vi "Drive Controller.vi"(8 "error in":errorcluster) -> ()   [LabVIEW 2020]
doc: "This VI executes continuously carrying out the current operation and responding to updates or new operation requests. It will often contain the timing or control code that is difficult to place directly in TeleOp. This VI generally opens all sensors and motors and isolates the rest of the robot code from knowing implementation details of how the operations are carried out."
uses:
  <vilib>/Rock Robotics/WPI/Framework/Completion Status.ctl
  Drive Setpoints.ctl
  Drive Operations.ctl
  Support Code/submodules/bordeaux-pathinator/Bordeaux/Types/Single Cmd Info.ctl
  <vilib>/picture/picture.llb/imagedata.ctl
  <vilib>/Rock Robotics/WPI/ThirdParty/Phoenix-LabVIEW/Motor Controller/Controls/CTRE_Phoenix_MotorControl_ControlMode.ctl
  <vilib>/Platform/TimedLoop/XDataNode/timing_clust.ctl
  <vilib>/Platform/TimedLoop/XDataNode/nitl_modes.ctl
  <vilib>/Platform/TimedLoop/XDataNode/wakeup.ctl
  <vilib>/Rock Robotics/WPI/ThirdParty/Phoenix-LabVIEW/CANCoder/Get/CTRE_Phoenix_CANcoder_GetSensorData.vi
  <vilib>/Platform/TimedLoop/XDataNode/XDataNode.xnode
  <vilib>/Platform/TimedLoop/XDataNode/XDNodeRunTimeDep.lvlib
  7c524804-90ba-49ae-a8d8-e902cfb15891.vi
  Framework/Robot Global Data.vi
  03237a54-0aa6-442f-88f7-9e8753c34860.vi
  829c4970-17fc-441a-8aa9-59a5cf39e87e.vi
panel:
  out "size(s)":i32
  in  "IMU Correction  2":bool=TRUE
  out "Waveform Chart":dbl(graph)
  out "output cluster 2":T1
  out "output cluster":T2
  in  "teleop imu":bool
  in  "RESET CANCODERS -- TEST":bool
  in  "IMU Correction":bool=TRUE
  out "offsets":cluster{dbl, dbl, dbl, dbl}
  in  "pod radius":dbl=1.166667
  in  "Interactive Values":T3
  in  "Buttons":cluster{"Execute Cmd":bool, "Abort Cmd":bool}
  out "Command Timing":cluster{"Start Time (ms)":u32, "Iterations":i32}
  out "Status":T7
  out "Current\nCmd":string
  # "Tip: The graph shows the motor setpoints. It may also be helpful to observe inputs and sensor values.\nYou may also want to display tuning or debugging controls."
  # "Interactive Command: You may fill in the settings for a command\nand schedule it with the Execute button. You can observe and abort\nany command while fine tuning the code for the controller."
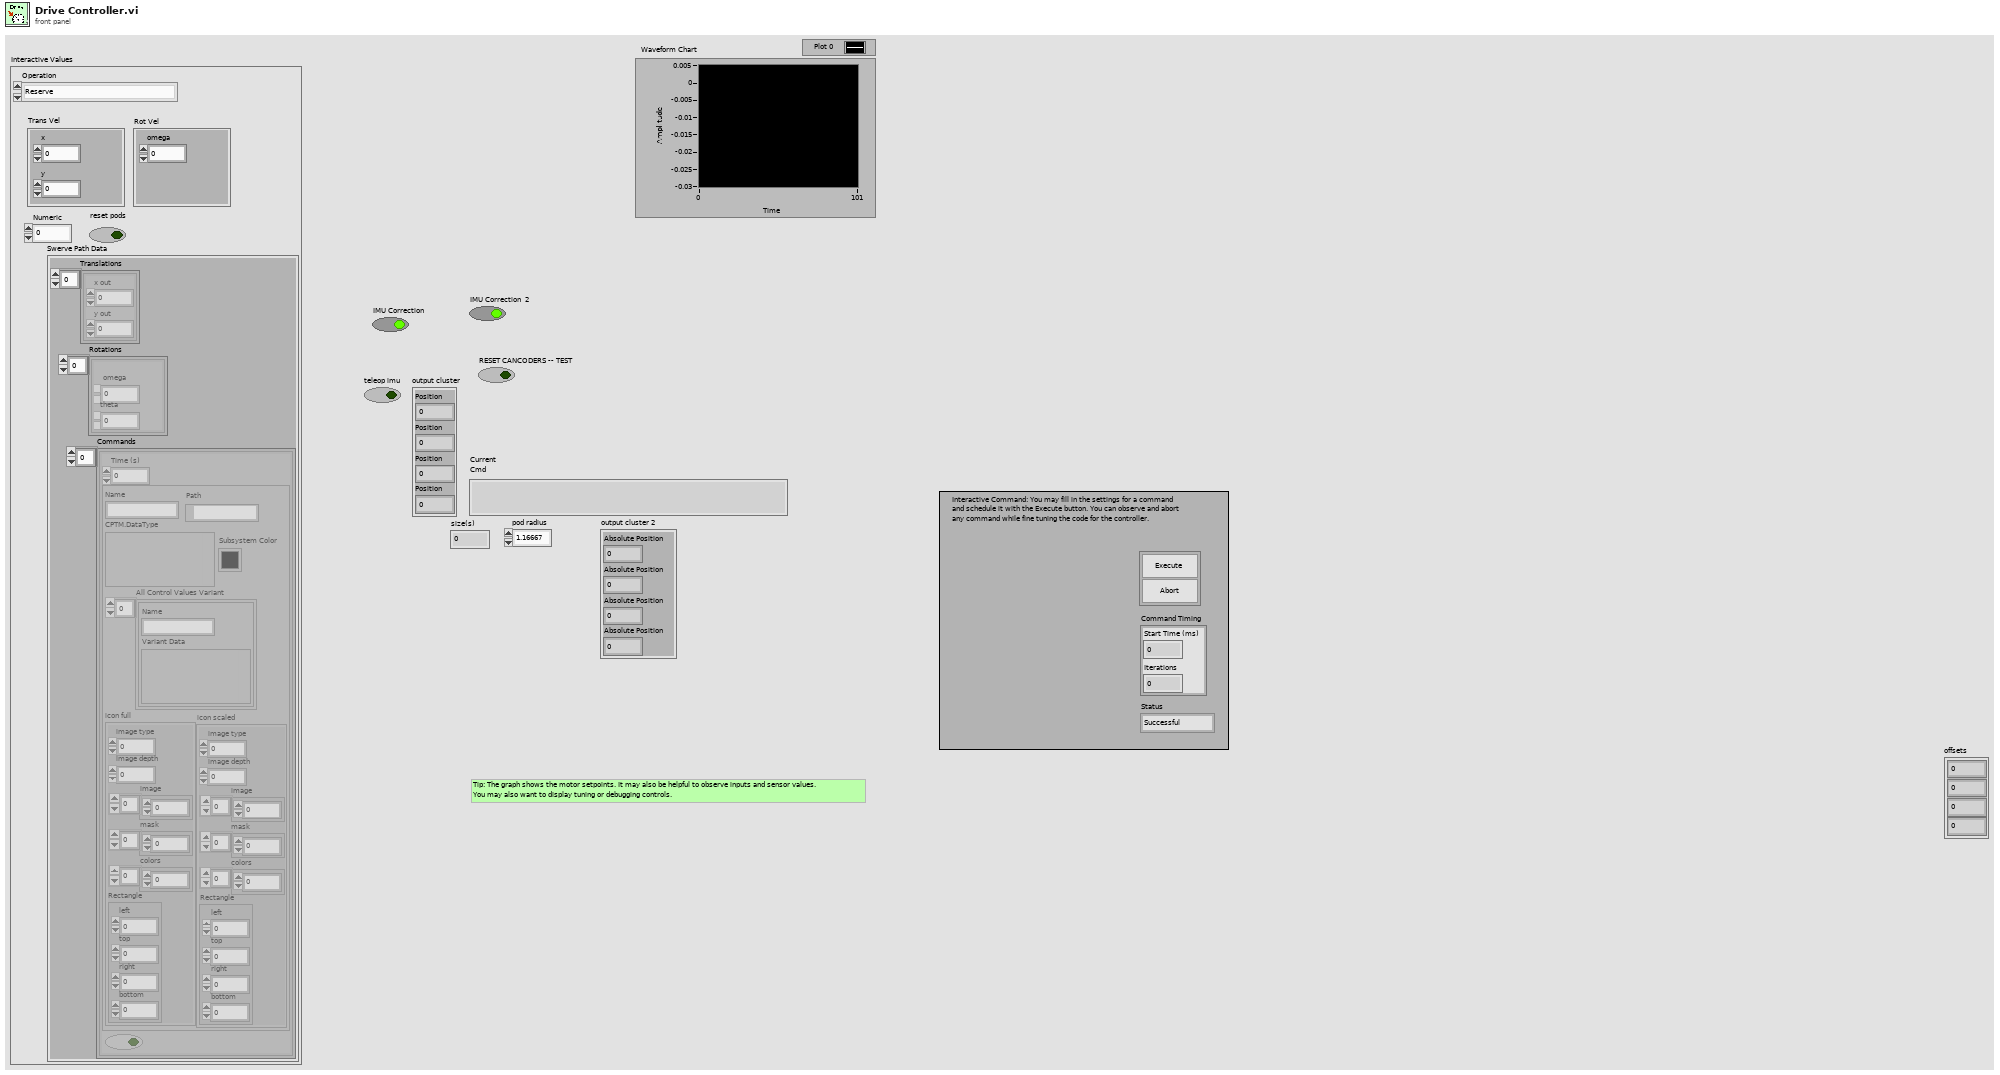
[diagram p1: front panel]
types:
  T1 = cluster{"Absolute Position":dbl, "Absolute Position":dbl, "Absolute Position":dbl, "Absolute Position":dbl}
  T2 = cluster{"Position":dbl, "Position":dbl, "Position":dbl, "Position":dbl}
  T3 = typedef "Drive Setpoints.ctl" = cluster{"Operation":T4, "Trans Vel":cluster{"x":dbl, "y":dbl}, "Rot Vel":cluster{"omega":dbl}, "Swerve Path Data":cluster{"Translations":cluster{"x out":dbl, "y out":dbl}[], "Rotations":cluster{"omega":dbl, "theta":dbl}[], "Commands":cluster{"Time (s)":dbl, T5, bool}[]}, "reset pods":bool, "Numeric":dbl}
  T4 = typedef "Drive Operations.ctl" = enum16{"Reserve", "Read Current", "Immediate", "Calibrate", "Play Path", "Immediate MM", "Set Schtuff"}
  T5 = typedef "Single Cmd Info.ctl" = cluster{"Name":string, "CPTM.DataType":variant, "All Control Values Variant":cluster{"Name":string, "Variant Data":variant}[], "icon full":T6, "icon scaled":T6, "Path":path, "Subsystem Color":u32}
  T6 = typedef "imagedata.ctl" = cluster{"image type":i32, "image depth":i32, "image":u8[], "mask":u8[], "colors":u32[], "Rectangle":cluster{"left":i16, "top":i16, "right":i16, "bottom":i16}}
  T7 = typedef "Completion Status.ctl" = enum16{"Successful", "Aborted", "Incomplete"}
  T8 = cluster{"LF ID":u8, "LB ID":u8, "RF ID":u8, "RB ID":u8}
  T9 = cluster{"LF radius":dbl[], "LB radius":dbl[], "RF radius":dbl[], "RB radius":dbl[]}
  T10 = typedef "Command Status Info.ctl" = cluster{"Name":string, "Status":T7, "notifier out":T11}
  T11 = typedef "Completion Notifier.ctl" = refnum<notifier>
  T12 = cluster{"SubSystem Data":T3, cluster{"Start Time (ms)":u32, "Iterations":i32}, cluster{"Command Info":T10, "Description":string, "Default Command":T3, "queue out":refnum<queue>, "Subsystem Name":string}}
  T13 = typedef "CTRE_Phoenix_MotorControl_BufferedTrajectoryPointStream_DeviceRef.ctl" = cluster{"Handle":u64, "Library Path":path}
  T14 = cluster{"BufferedTrajectoryPointStream_DevRef":T13, "BufferedTrajectoryPointStream_DevRef":T13, "BufferedTrajectoryPointStream_DevRef":T13, "BufferedTrajectoryPointStream_DevRef":T13}
  T15 = typedef "WPI_MotorControlDeviceRef.ctl" = cluster{"DeviceStatus":errorcluster, "Type":T16, "PWM":cluster{"PWM Channel":T17, "DeadBand":T18}, "CAN":cluster{"Device Number":u8, "SetOutput VI Ref":variant, "GetOutput VI Ref":variant, "Enable VI Ref":variant, "Disable VI Ref":variant, "Data":variant}, "Invert":bool, "DIO PWM":cluster{"PWM \"Enable\" Channel":T17, "DIOChannel":T19, "PWM Rate":dbl}}
  T16 = typedef "WPI_MotorControlType.ctl" = enum16{"PWM", "CAN", "DIO PWM"}
  T17 = typedef "FPGA_DIOPWMChannel.ctl" = enum8{"PWM 0", "PWM 1", "PWM 2", "PWM 3", "PWM 4", "PWM 5", "PWM 6", "PWM 7", "PWM 8", "PWM 9", "PWM MXP 0", "PWM MXP 1", "PWM MXP 2", "PWM MXP 3", "PWM MXP 4", "PWM MXP 5", "PWM MXP 6", "PWM MXP 7", "PWM MXP 8", "PWM MXP 9", "Invalid"}
  T18 = typedef "WPI_PWMDeadband.ctl" = cluster{"Name":string, "maxPositivePwm":i32, "minPositivePwm":i32, "centerPwm":i32, "maxNegativePwm":i32, "minNegativePwm":i32, "angularRange":u16}
  T19 = typedef "FPGA_DIOChannel.ctl" = enum8{"DIO 0", "DIO 1", "DIO 2", "DIO 3", "DIO 4", "DIO 5", "DIO 6", "DIO 7", "DIO 8", "DIO 9", "DIO MXP 0", "DIO MXP 1", "DIO MXP 2", "DIO MXP 3", "DIO MXP 4", "DIO MXP 5", "DIO MXP 6", "DIO MXP 7", "DIO MXP 8", "DIO MXP 9", "DIO MXP 10", "DIO MXP 11", "DIO MXP 12", "DIO MXP 13", "DIO MXP 14", "DIO MXP 15", "SPI Port CS1", "SPI Port CS2", "SPI Port CS3", "SPI Port MISO", "SPI Port MOSI", "Invalid"}
  T20 = cluster{"PhoenixMotorControlDevRef":T15, "PhoenixMotorControlDevRef":T15, "PhoenixMotorControlDevRef":T15, "PhoenixMotorControlDevRef":T15}
  T21 = typedef "ADIS16470 Device Reference.ctl" = cluster{"DevStatus":errorcluster, "Hardware Config":T22, "Calibration Complete":refnum<notifier>, "Status Reference":refnum<data-value>, "Position Reference":refnum<data-value>, "Velocity Reference":refnum<data-value>, "Sychronous Process VI":T25, "Cmd FIFO":refnum<k33>, "Source":T26, "Data FIFO":refnum<k33>, "Calibration Time (ms)":u32}
  T22 = typedef "ADIS16470 Hardware Configuration.ctl" = cluster{"SPI Clock Rate (Hz)":dbl, "IMU SPI Mode (3)":T23, "IMU Reset Pin":T19, "IMU SPI Bus":T24, "IMU Data Ready Pin":T19, "Stall Config":cluster{"Pow2BytesPerRead":u8, "StallTicks":u16, "CsToSclkTicks":u8}}
  T23 = typedef "WPI_SPIMode.ctl" = enum16{"Mode 0 (Clk Idle Low,Sample on Leading)", "Mode 1 (Clk Idle Low,Sample on Trailing)", "Mode 2 (Clk Idle High,Sample on Leading)", "Mode 3 (Clk Idle High,Sample on Trailing)"}
  T24 = typedef "spi_bus.ctl" = enum16{"SPI On-Board, CS0", "SPI On-Board, CS1", "SPI On-Board, CS2", "SPI On-Board, CS3", "SPI MXP", "Invalid"}
  T25 = typedef "ADIS16470 Process.ctl" = refnum<vi>
  T26 = typedef "FPGA_CounterEncoderSourceConvertionLVSourceType.ctl" = cluster{"DevStatus":errorcluster, "AnalogTriggerMode?":bool, "DigitalMode":cluster{"DIO Channel":T27}, "AnalogTriggerMode":cluster{"AnalogTriggerIndex":T28, "OutputType":T29}}
  T27 = typedef "FPGA_DIODigitalSourceChannel.ctl" = enum8{"DIO 0", "DIO 1", "DIO 2", "DIO 3", "DIO 4", "DIO 5", "DIO 6", "DIO 7", "DIO 8", "DIO 9", "DIO MXP 0", "DIO MXP 1", "DIO MXP 2", "DIO MXP 3", "DIO MXP 4", "DIO MXP 5", "DIO MXP 6", "DIO MXP 7", "DIO MXP 8", "DIO MXP 9", "DIO MXP 10", "DIO MXP 11", "DIO MXP 12", "DIO MXP 13", "DIO MXP 14", "DIO MXP 15", "SPI Port CS1", "SPI Port CS2", "SPI Port CS3", "SPI Port MISO", "SPI Port MOSI", "Disabled"}
  T28 = typedef "FPGA_AnalogTriggerIndex.ctl" = enum8{"Trig 0", "Trig 1", "Trig 2", "Trig 3", "Trig 4", "Trig 5", "Trig 6", "Trig 7", "Invalid"}
  T29 = typedef "FPGA_AnalogTriggerOutType.ctl" = enum16{"InWindow", "TriggerState", "Rising", "Falling"}
  T30 = typedef "CTRE_Phoenix_CANcoder_DeviceRef.ctl" = cluster{"DeviceStatus":errorcluster, "Device Number":u8, "Handle":u64, "UsageFrame":u32, "Library Path":path}
  T31 = cluster{"CTRE_CANcoder_DeviceRef":T30, "CTRE_CANcoder_DeviceRef":T30, "CTRE_CANcoder_DeviceRef":T30, "CTRE_CANcoder_DeviceRef":T30}
  T32 = typedef "XDNodeRunTimeDep.lvlib/timing_clust.ctl" = cluster{"Expected End [f-1]":u64, "Actual End [f-1]":u64, "Finished Late? [f-1]":bool, "Expected End [i-1]":u64, "Actual End [i-1]":u64, "Finished Late? [i-1]":bool, "Expected Start [i]":u64, "Actual Start [i]":u64, "Expected Start [f]":u64, "Actual Start [f]":u64, "Source Name":string, "Structure Name":string, "Period":i64, "Deadline":i64, "Offset":i64, "Start":i64, "Priority":i32, "Timeout":i32, "Mode":T33, "Wakeup Reason":T34, "Error":errorcluster, "Source Type":string, "Secondary Source Type":string, "Global End Time":u64, "Global Start Time":u64, "Frame Duration":u64, "Iteration Duration":u64, "Assigned CPU":i32, "I/O Scan Engine Mode":u32}
  T33 = typedef "XDNodeRunTimeDep.lvlib/nitl_modes.ctl" = enum32{"No Change", "Process missed periods, maintain original phase", "Discard missed periods, maintain original phase", "Process missed periods, ignore original phase", "Discard missed periods, ignore original phase"}
  T34 = typedef "XDNodeRunTimeDep.lvlib/wakeup.ctl" = enum32{"Normal", "Aborted", "Asynchronous wakeup", "Timing source error", "Timed loop error", "Timeout"}
  T35 = cluster{"Translations":cluster{"x out":dbl, "y out":dbl}[], "Rotations":cluster{"omega":dbl, "theta":dbl}[], "Commands":cluster{"Time (s)":dbl, T5, bool}[]}
  T36 = typedef "CTRE_Phoenix_MotorControl_ControlMode.ctl" = u16
  T37 = typedef "ADIS16470 Data.ctl" = cluster{"XAngle":dbl, "YAngle":dbl, "ZAngle":dbl}
  T38 = cluster{"Position (degrees)":dbl, "Position (degrees)":dbl, "Position (degrees)":dbl, "Position (degrees)":dbl}
  T39 = cluster{"Theta":dbl, "Theta":dbl, "Theta":dbl, "Theta":dbl}
  T40 = cluster{"Velocity":dbl, "Velocity":dbl, "Velocity":dbl, "Velocity":dbl}
  T41 = cluster{"angle out":dbl, "angle out":dbl, "angle out":dbl, "angle out":dbl}
  T42 = cluster{"SubSystem Data":T3, cluster{"Start Time (ms)":u32, "Iterations":i32}, "Default Command Arguments":cluster{"Command Info":T10, "Description":string, "Default Command":T3, "queue out":refnum<queue>, "Subsystem Name":string}}
  T43 = typedef "numlock.ctl" = cluster{"tdms file out":refnum<k34>, "Default log level (info)":enum16{"trace", "debug", "info", "warn", "error"}}
  T44 = cluster{u32, "Trans Vel":cluster{"x":dbl, "y":dbl}}
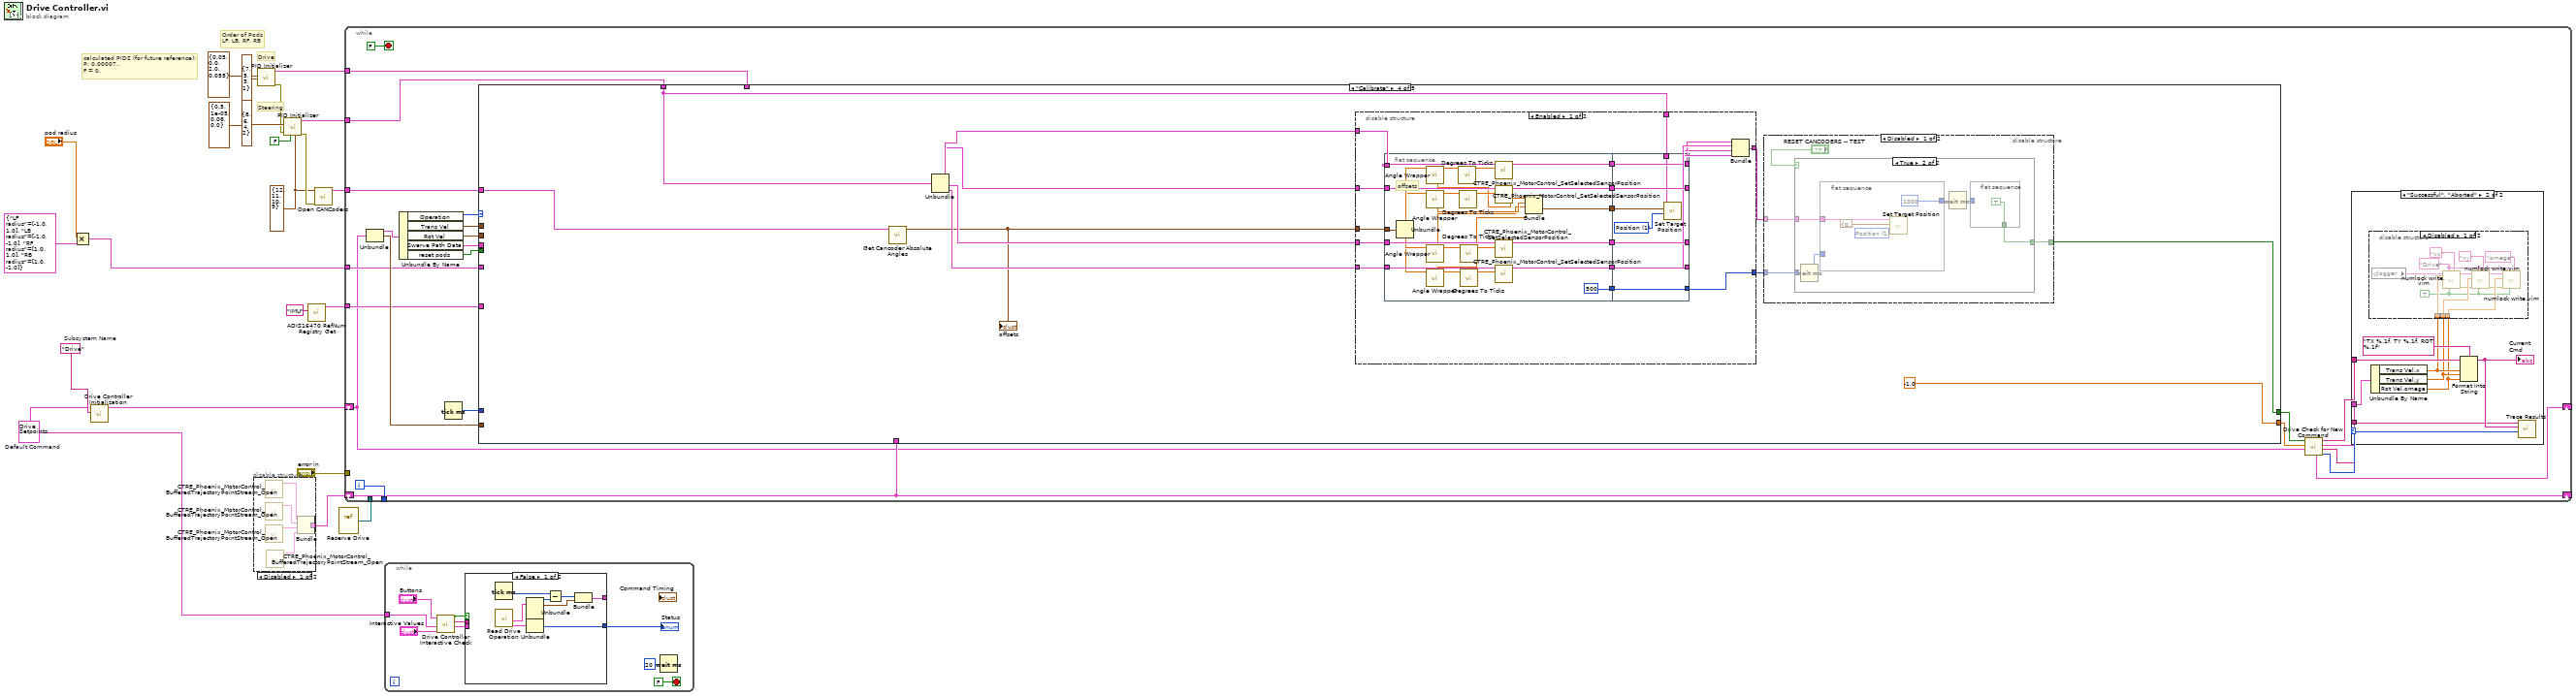
[diagram p0: block diagram]
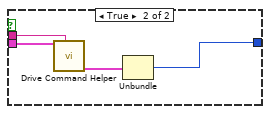
[diagram p3: hidden frame]
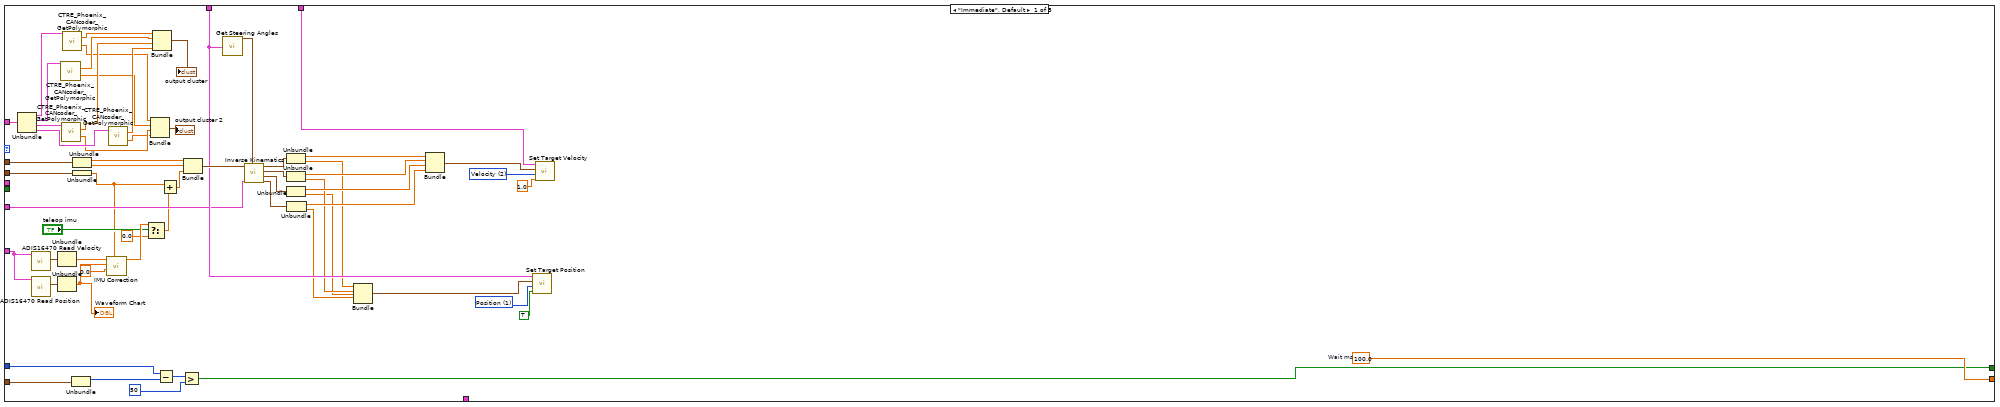
[diagram p6: hidden frame]
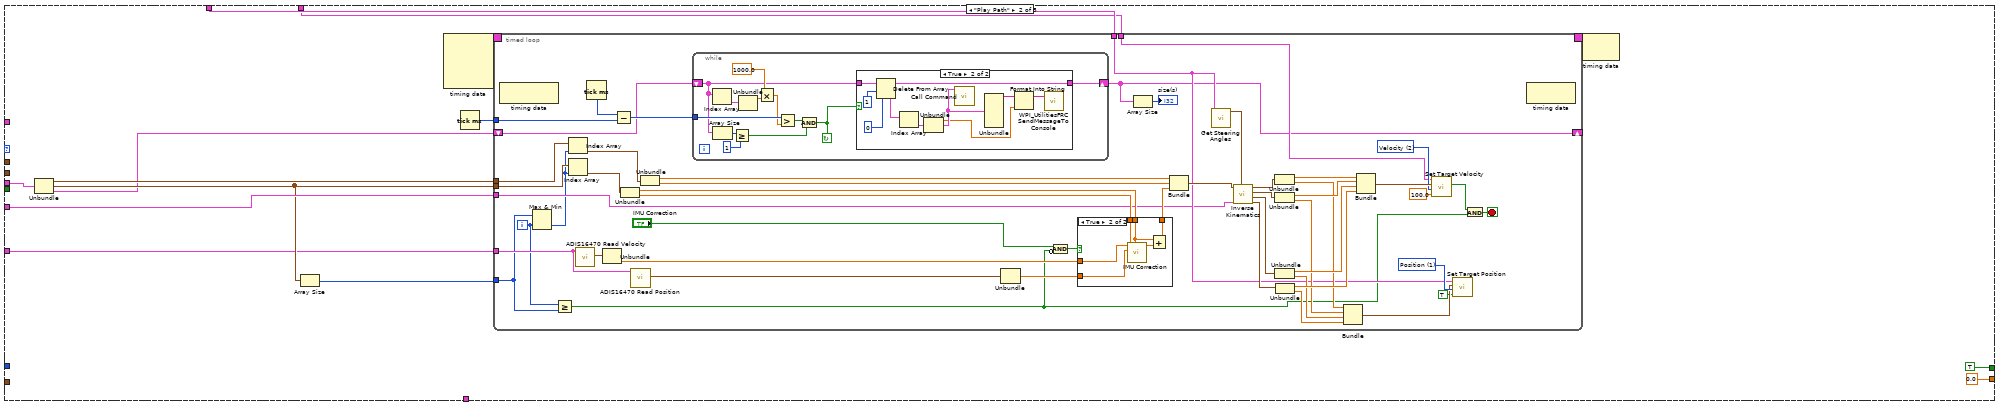
[diagram p7: hidden frame]
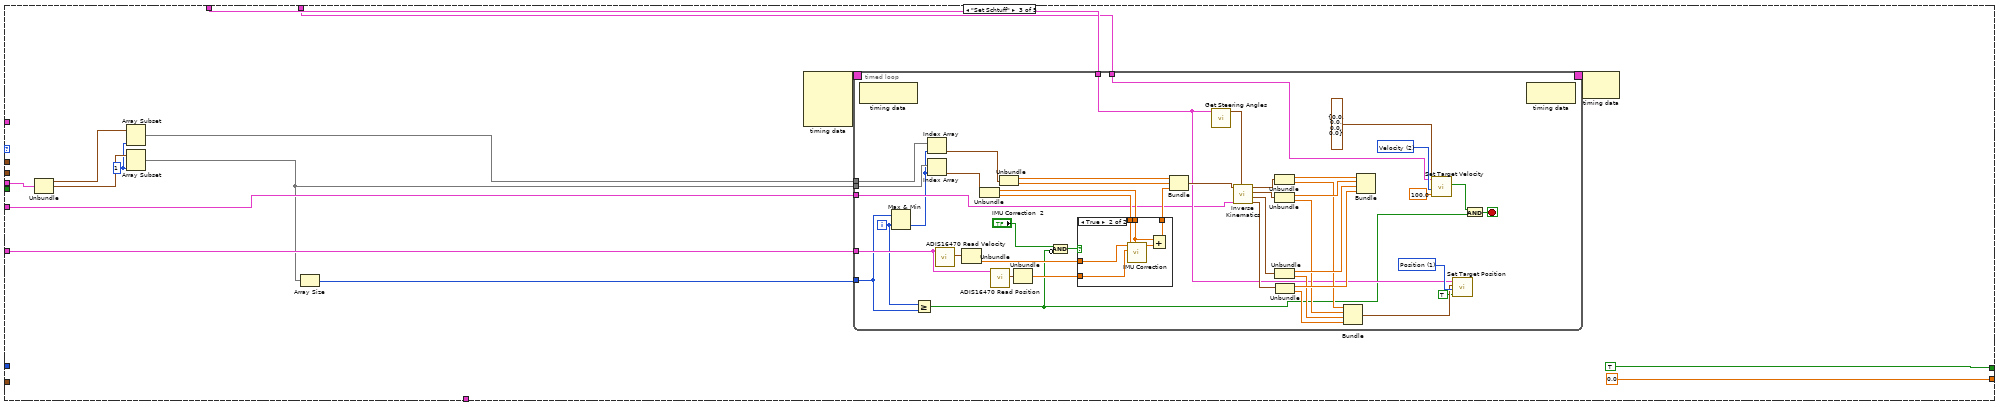
[diagram p10: hidden frame]
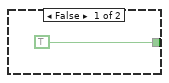
[diagram p13: hidden frame]
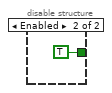
[diagram p14: hidden frame]
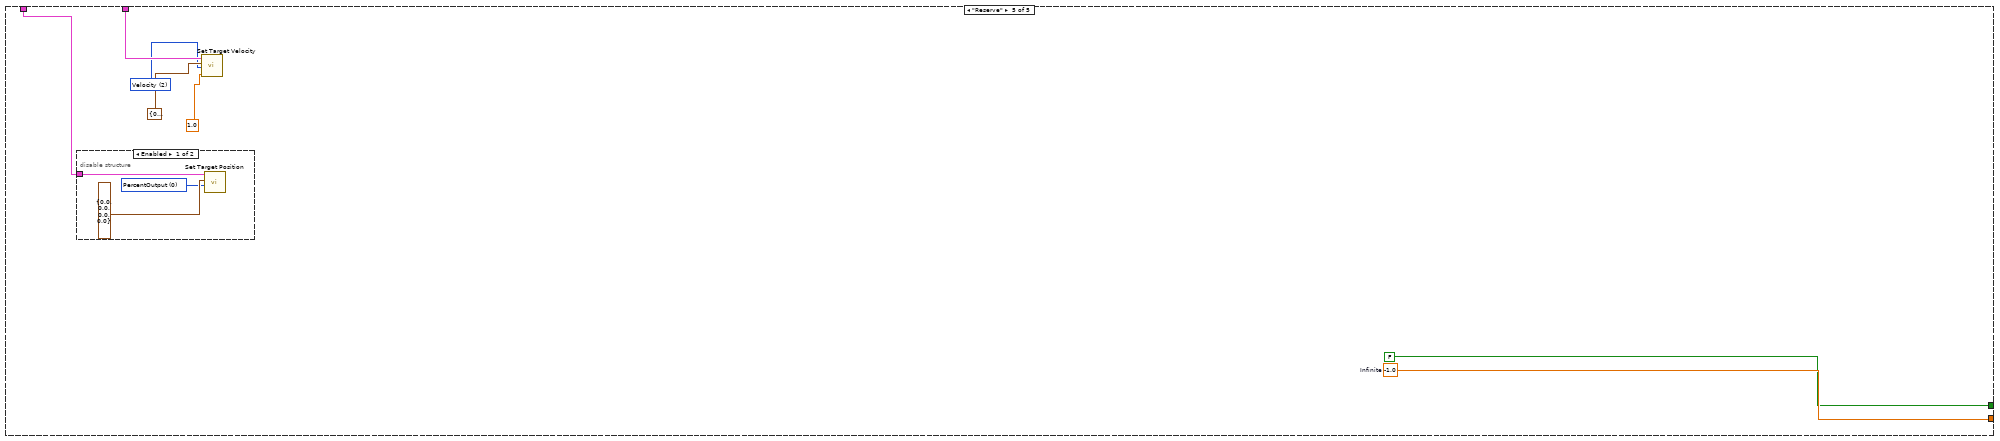
[diagram p15: hidden frame]
diagram:
  w1 = T8 {"LF ID"=12, "LB ID"=11, "RF ID"=10, "RB ID"=9} ("CANCoder Can IDs")
  w18 = T3 {"Operation"=enum."Reserve", "Trans Vel"={"x"=0.0, "y"=0.0}, "Rot Vel"={"omega"=0.0}, "Swerve Path Data"={"Translations"=[], "Rotations"=[], "Commands"=[]}, "reset pods"=FALSE, "Numeric"=0.0}  # Default Command
  w22 = "Drive"  # Subsystem Name
  # "calculated PIDS (for future reference): \nP: 0.00007..\nF = 0."
  # "Order of Pods\nLF, LB, RF, RB"
  # "Steering"
  # "Drive"
  n1 = Multiply(x="pod radius", y=T9 {"LF radius"=[-1.0, 1.0], "LB radius"=[-1.0, -1.0], "RF radius"=[1.0, 1.0], "RB radius"=[1.0, -1.0]} ("Radii")) -> (x*y=w15:T9)
  n2 = call "Drive Controller Initialization.vi"("Subsystem Name"=w22, "Default Command"=w18) -> ("Current Command"=w20:T12)  [unwired: 9 in]
  n3 = disable-structure shown="Disabled" {
    disable-tunnel: [w23 _] -> w6
    frame Disabled {
      n4 = call <vilib>:"CTRE_Phoenix_MotorControl_BufferedTrajectoryPointStream_Open.vi"() -> ("BufferedTrajectoryPointStream_DevRef"=w27:T13)  [unwired: 10 in, 1 out]
      n5 = call <vilib>:"CTRE_Phoenix_MotorControl_BufferedTrajectoryPointStream_Open.vi"() -> ("BufferedTrajectoryPointStream_DevRef"=w26:T13)  [unwired: 10 in, 1 out]
      n6 = call <vilib>:"CTRE_Phoenix_MotorControl_BufferedTrajectoryPointStream_Open.vi"() -> ("BufferedTrajectoryPointStream_DevRef"=w25:T13)  [unwired: 10 in, 1 out]
      n7 = call <vilib>:"CTRE_Phoenix_MotorControl_BufferedTrajectoryPointStream_Open.vi"() -> ("BufferedTrajectoryPointStream_DevRef"=w24:T13)  [unwired: 10 in, 1 out]
      n8 = Bundle("BufferedTrajectoryPointStream_DevRef"=w27, "BufferedTrajectoryPointStream_DevRef"=w26, "BufferedTrajectoryPointStream_DevRef"=w25, "BufferedTrajectoryPointStream_DevRef"=w24) -> (w23:T14)  [unwired: 1 in]
    }
    frame Enabled {
    }
  }
  n9 = call "PID Initializer.vi"("PIDF"=cluster{"P":dbl, "I":dbl, "D":dbl, "F":dbl} {"P"=0.05, "I"=0.0, "D"=2.0, "F"=0.055} ("drive PIDF"), "Can IDs"=T8 {"LF ID"=7, "LB ID"=5, "RF ID"=3, "RB ID"=1}) -> ("error out"=w10:errorcluster, "Motors"=w14:T20)  [unwired: 8 in]
  n10 = call "PID Initializer.vi"("CANCoder Can IDs"=w1, "Cancoder????"=FALSE, "error in"=w10, "PIDF"=cluster{"P":dbl, "I":dbl, "D":dbl, "F":dbl} {"P"=0.5, "I"=1e-05, "D"=0.08, "F"=0.0} ("steer PIDF"), "Can IDs"=T8 {"LF ID"=8, "LB ID"=6, "RF ID"=4, "RB ID"=2}) -> ("error out"=w2:errorcluster, "Motors"=w13:T20)  [unwired: 5 in]
  n11 = call "ADIS16470 RefNum Registry Get.vi"("refnum name"="IMU") -> ("ADIS16470DevRef out"=w7:T21)  [unwired: 9 in, 1 out]
  n12 = call "Open CANCoders.vi"("error in"=w2, "CANCoder Can IDs"=w1) -> ("output cluster"=w9:T31)  [unwired: 9 in]
  n13 = vi-ref "Reserve Drive.vi"() -> (w19:refnum<vi>)
  n14 = while {
    shift-right: [w43] -> _
    shift-left: w20 -> [w28]
    tunnel: [w50] -> _
    tunnel: "error in" -> [_]
    tunnel: w19 -> [_]
    tunnel: w15 -> [w36]
    tunnel: w14 -> [w35]
    tunnel: w13 -> [w34]
    tunnel: w9 -> [w33]
    tunnel: w7 -> [w31]
    shift-right: [w29] -> _
    shift-left: w6 -> [w29]
    i -> [w50]
    stop <- FALSE stop-if-true
    n15 = Unbundle(w28) -> ("SubSystem Data"=w49:T3, w37:cluster{"Start Time (ms)":u32, "Iterations":i32})  [unwired: 1 out]
    n16 = Unbundle By Name(w49) -> ("Operation"=w48:T4, "Trans Vel"=w47:cluster{"x":dbl, "y":dbl}, "Rot Vel"=w46:cluster{"omega":dbl}, "Swerve Path Data"=w32:T35, "reset pods"=w30:bool)
    n17 = Tick Count (ms)() -> (millisecond timer value=w45:u32)
    n18 = case shown="\"Calibrate\"" w48 {
      tunnel: [w134 0.0 ("Infinite") 0.0 ("Infinite") -1.0 ("Infinite") w388] -> w42
      tunnel: [w132 TRUE ("ignore previous (F)") TRUE ("ignore previous (F)") w314 FALSE ("ignore previous (F)")] -> w41
      tunnel: w37 -> [w131 _ _ _ _]
      tunnel: w47 -> [w122 _ _ _ _]
      tunnel: w46 -> [w121 _ _ _ _]
      tunnel: w45 -> [w133 _ _ _ _]
      tunnel: w36 -> [w105 w140 w241 _ _]
      tunnel: w35 -> [w117 w143 w244 _ w385]
      tunnel: w34 -> [w115 w144 w245 w312 w383]
      tunnel: w33 -> [w96 _ _ w313 _]
      tunnel: w32 -> [_ w146 w246 _ _]
      tunnel: w31 -> [w78 w137 w239 _ _]
      tunnel: w30 -> [_ _ _ _ _]
      tunnel: w29 -> [_ _ _ _ _]
      frame "Immediate", Default {
        w134 = 100.0  # Wait ms
        w110 = T36 1 items=["PercentOutput"=0, "Position"=1, "Velocity"=2, "Current"=3, "Follower"=5, "MotionProfile"=6, "MotionMagic"=7, "MotionProfileArc"=10, "Disabled"=15] ("Control Mode")
        w111 = T36 2 items=["PercentOutput"=0, "Position"=1, "Velocity"=2, "Current"=3, "Follower"=5, "MotionProfile"=6, "MotionMagic"=7, "MotionProfileArc"=10, "Disabled"=15] ("Control Mode")
        n19 = Unbundle(w96) -> ("CTRE_CANcoder_DeviceRef"=w95:T30, "CTRE_CANcoder_DeviceRef"=w94:T30, "CTRE_CANcoder_DeviceRef"=w93:T30, "CTRE_CANcoder_DeviceRef"=w92:T30)
        n20 = call "ADIS16470 Read Velocity.vi"("ADIS16470DevRef"=w78) -> ("ADIS16470 Value"=w103:T37)  [unwired: 7 in, 3 out]
        n21 = call "ADIS16470 Read Position.vi"("ADIS16470DevRef"=w78) -> ("ADIS16470 Value"=w79:T37)  [unwired: 7 in, 3 out]
        n22 = Unbundle(w103) -> ("YAngle"=w102:dbl)  [unwired: 2 out]
        n23 = Unbundle(w79) -> ("YAngle"=w76:dbl)  [unwired: 2 out]
        "Waveform Chart" <- w76
        n24 = call-poly <vilib>:"CTRE_Phoenix_CANcoder_GetPolymorphic.vi"("CTRE_CANcoder_DeviceRef"=w94) -> ("Position"=w90:dbl, "Absolute Position"=w85:dbl)  [unwired: 10 in, 3 out]
        n25 = call-poly <vilib>:"CTRE_Phoenix_CANcoder_GetPolymorphic.vi"("CTRE_CANcoder_DeviceRef"=w93) -> ("Position"=w89:dbl, "Absolute Position"=w84:dbl)  [unwired: 10 in, 3 out]
        n26 = call-poly <vilib>:"CTRE_Phoenix_CANcoder_GetPolymorphic.vi"("CTRE_CANcoder_DeviceRef"=w95) -> ("Position"=w91:dbl, "Absolute Position"=w86:dbl)  [unwired: 10 in, 3 out]
        n27 = Unbundle(w131) -> ("Start Time (ms)"=w112:u32)  [unwired: 1 out]
        n28 = Unbundle(w122) -> ("x"=w120:dbl, "y"=w119:dbl)
        n29 = Unbundle(w121) -> ("omega"=w80:dbl)
        n30 = call "IMU Correction.vi"("omega"=w80, "Heading Setpoint"=0.0, "theta"=w76, "measured angle"=w102) -> ("Difference"=w101:dbl)  [unwired: 7 in]
        n31 = call-poly <vilib>:"CTRE_Phoenix_CANcoder_GetPolymorphic.vi"("CTRE_CANcoder_DeviceRef"=w92) -> ("Position"=w88:dbl, "Absolute Position"=w83:dbl)  [unwired: 10 in, 3 out]
        n32 = Select(t=w101, s="teleop imu", f=0.0) -> (s? t:f=w104:dbl)
        n33 = Bundle("Absolute Position"=w86, "Absolute Position"=w85, "Absolute Position"=w84, "Absolute Position"=w83) -> (→"output cluster 2":T1)  [unwired: 1 in]
        n34 = Bundle("Position"=w91, "Position"=w90, "Position"=w89, "Position"=w88) -> (→"output cluster":T2)  [unwired: 1 in]
        n35 = Subtract(x=w133, y=w112) -> (x-y=w113:u32)
        n36 = Add(x=w80, y=w104) -> (x+y=w75:dbl)
        n37 = Greater?(x=w113, y=u8 50 ("Left Motor")) -> (0:w132:bool)
        n38 = Bundle("x"=w120, "y"=w119, w75) -> (w118:cluster{"x":dbl, "y":dbl, dbl})  [unwired: 1 in]
        n39 = call "Get Steering Angles.vi"("Input Steering"=w115) -> ("Steering Angles (deg)"=w81:T38)  [unwired: 10 in]
        n40 = call "Inverse Kinematics.vi"("Current Pod Steering (deg)"=w81, "Radii (ft)"=w105, "Target Velocity (ft/s and deg/s)"=w118) -> ("RB Pod Setpoint (ft/s and deg/s)"=w127:cluster{"Velocity":dbl, "Theta":dbl}, "RF Pod Setpoint (ft/s and deg/s)"=w128:cluster{"Velocity":dbl, "Theta":dbl}, "LB Pod Setpoint (ft/s and deg/s)"=w129:cluster{"Velocity":dbl, "Theta":dbl}, "LF Pod Setpoint (ft/s and deg/s)"=w130:cluster{"Velocity":dbl, "Theta":dbl})  [unwired: 2 in, 3 out]
        n41 = Unbundle(w130) -> ("Velocity"=w126:dbl, "Theta"=w109:dbl)
        n42 = Unbundle(w129) -> ("Velocity"=w125:dbl, "Theta"=w108:dbl)
        n43 = Unbundle(w128) -> ("Velocity"=w124:dbl, "Theta"=w107:dbl)
        n44 = Unbundle(w127) -> ("Velocity"=w123:dbl, "Theta"=w106:dbl)
        n45 = Bundle("Theta"=w109, "Theta"=w108, "Theta"=w107, "Theta"=w106) -> (w97:T39)  [unwired: 1 in]
        n46 = Bundle("Velocity"=w126, "Velocity"=w125, "Velocity"=w124, "Velocity"=w123) -> (w116:T40)  [unwired: 1 in]
        n47 = call "Set Target Position.vi"("conv to ticks?"=TRUE, "Control Mode"=w110, "Input (deg)"=w97, "Swerve motors"=w115) -> ()  [unwired: 7 in, 1 out]
        n48 = call "Set Target Velocity.vi"("epsilon"=1.0, "Control Mode"=w111, "Input (ft/s)"=w116, "Swerve motors"=w117) -> ()  [unwired: 6 in, 2 out]
      }
      frame "Play Path" {
        n49 = Unbundle(w146) -> ("Translations"=w145:cluster{"x out":dbl, "y out":dbl}[], "Rotations"=w139:cluster{"omega":dbl, "theta":dbl}[], "Commands"=w136:cluster{"Time (s)":dbl, T5, bool}[])
        n50 = Array Size(array=w139) -> (size(s)=w138:i32)
        n51 = node-c288() -> (w148:T32)  [unwired: 4 in]
        n52 = Tick Count (ms)() -> (millisecond timer value=w135:u32)
        n53 = timed-loop {
          timing: w148 -> [_]
          timing-out: [_] -> w147
          tunnel: w145 -> [w167]
          tunnel: w139 -> [w166]
          tunnel: w144 -> [w181]
          tunnel: w143 -> [w182]
          tunnel: w140 -> [w168]
          tunnel: w138 -> [w161]
          tunnel: w137 -> [w172]
          tunnel: w135 -> [w153]
          shift-right: [w150] -> _
          shift-left: w136 -> [w151]
          i -> [w162]
          stop <- w158 stop-if-true
          w184 = T36 1 items=["PercentOutput"=0, "Position"=1, "Velocity"=2, "Current"=3, "Follower"=5, "MotionProfile"=6, "MotionMagic"=7, "MotionProfileArc"=10, "Disabled"=15] ("Control Mode")
          w185 = T36 2 items=["PercentOutput"=0, "Position"=1, "Velocity"=2, "Current"=3, "Follower"=5, "MotionProfile"=6, "MotionMagic"=7, "MotionProfileArc"=10, "Disabled"=15] ("Control Mode")
          n54 = node-c288() -> ()  [unwired: 1 in, 1 out]
          n55 = Max & Min(x=w161, y=w162) -> (min(x,y)=w159:i32)  [unwired: 1 out]
          n56 = Greater Or Equal?(x=w162, y=w161) -> (x >= y?=w156:bool)
          n57 = Index Array(array=w167, index=w159) -> (element=w165:cluster{"x out":dbl, "y out":dbl})
          n58 = Index Array(array=w166, index=w159) -> (element=w164:cluster{"omega":dbl, "theta":dbl})
          n59 = call "ADIS16470 Read Velocity.vi"("ADIS16470DevRef"=w172) -> ("ADIS16470 Value"=w177:T37)  [unwired: 7 in, 3 out]
          n60 = Tick Count (ms)() -> (millisecond timer value=w154:u32)
          n61 = Unbundle(w177) -> ("ZAngle"=w174:dbl)  [unwired: 2 out]
          n62 = Subtract(x=w154, y=w153) -> (x-y=w152:u32)
          n63 = Unbundle(w164) -> ("omega"=w179:dbl, "theta"=w173:dbl)
          n64 = call "ADIS16470 Read Position.vi"("ADIS16470DevRef"=w172) -> ("ADIS16470 Value"=w171:T37)  [unwired: 7 in, 3 out]
          n65 = Unbundle(w165) -> ("x out"=w175:dbl, "y out"=w176:dbl)
          n66 = while {
            tunnel: w152 -> [w210]
            shift-right: [w209] -> w150
            shift-left: w151 -> [w205]
            stop <- w200 continue-if-true
            n67 = Index Array(array=w205) -> (element=w211:cluster{"Time (s)":dbl, T5, bool})  [unwired: 1 in]
            n68 = Array Size(array=w205) -> (size(s)=w204:i32)
            n69 = Greater Or Equal?(x=w204, y=1) -> (x >= y?=w202:bool)
            n70 = Unbundle(w211) -> ("Time (s)"=w208:dbl)  [unwired: 2 out]
            n71 = Multiply(x=1000.0, y=w208) -> (x*y=w206:dbl)
            n72 = Greater?(x=w210, y=w206) -> (0:w201:bool)
            n73 = And(x=w201, y=w202) -> (x .and. y?=w200:bool)
            n74 = case shown="True" w200 {
              tunnel: w205 -> [w212 w222]
              tunnel: [w212 w220] -> w209
              frame False {
              }
              frame True {
                n75 = Delete From Array(array=w222, length=1, index=0) -> (deleted portion=w219:cluster{"Time (s)":dbl, T5, bool}[], array with subset deleted=w220:cluster{"Time (s)":dbl, T5, bool}[])
                n76 = Index Array(array=w219) -> (element=w218:cluster{"Time (s)":dbl, T5, bool})  [unwired: 1 in]
                n77 = Unbundle(w218) -> ("Time (s)"=w214:dbl, w217:T5)  [unwired: 1 out]
                n78 = call "Call Command.vi"("Command"=w217) -> ()  [unwired: 11 in]
                n79 = Unbundle(w217) -> ("Name"=w215:string)  [unwired: 6 out]
                n80 = Format Into String(initial string=w215, w214) -> (resulting string=w213:string)  [unwired: 2 in, 1 out]
                n81 = call <vilib>:"WPI_UtilitiesFRC SendMessageToConsole.vi"("Message"=w213) -> ()  [unwired: 14 in, 1 out]
              }
            }
          }
          n82 = Unbundle(w171) -> ("YAngle"=w170:dbl)  [unwired: 2 out]
          n83 = Compound Arithmetic op=AND("IMU Correction", invert w156) -> (w155:bool)
          n84 = case shown="True" w155 {
            tunnel: w174 -> [_ w229]
            tunnel: w179 -> [w223 w227]
            tunnel: [w223 w226] -> w178
            tunnel: w173 -> [_ w225]
            tunnel: w170 -> [_ w224]
            frame False {
            }
            frame True {
              n85 = call "IMU Correction.vi"("omega"=w227, "Heading Setpoint"=w225, "theta"=w224, "measured angle"=w229) -> ("Difference"=w228:dbl)  [unwired: 7 in]
              n86 = Add(x=w227, y=w228) -> (x+y=w226:dbl)
            }
          }
          n87 = Array Size(array=w150) -> (size(s)=→"size(s)":i32)
          n88 = Bundle("x out"=w175, "y out"=w176, "omega"=w178) -> (w183:cluster{"x out":dbl, "y out":dbl, "omega":dbl})  [unwired: 1 in]
          n89 = call "Get Steering Angles.vi"("Input Steering"=w181) -> ("Steering Angles (deg)"=w186:T38)  [unwired: 10 in]
          n90 = call "Inverse Kinematics.vi"("Current Pod Steering (deg)"=w186, "Radii (ft)"=w168, "Target Velocity (ft/s and deg/s)"=w183) -> ("RB Pod Setpoint (ft/s and deg/s)"=w196:cluster{"Velocity":dbl, "Theta":dbl}, "RF Pod Setpoint (ft/s and deg/s)"=w197:cluster{"Velocity":dbl, "Theta":dbl}, "LB Pod Setpoint (ft/s and deg/s)"=w198:cluster{"Velocity":dbl, "Theta":dbl}, "LF Pod Setpoint (ft/s and deg/s)"=w199:cluster{"Velocity":dbl, "Theta":dbl})  [unwired: 2 in, 3 out]
          n91 = Unbundle(w199) -> ("Velocity"=w195:dbl, "Theta"=w191:dbl)
          n92 = Unbundle(w198) -> ("Velocity"=w194:dbl, "Theta"=w190:dbl)
          n93 = Unbundle(w197) -> ("Velocity"=w193:dbl, "Theta"=w189:dbl)
          n94 = Unbundle(w196) -> ("Velocity"=w192:dbl, "Theta"=w188:dbl)
          n95 = Bundle("Theta"=w191, "Theta"=w190, "Theta"=w189, "Theta"=w188) -> (w180:T39)  [unwired: 1 in]
          n96 = Bundle("Velocity"=w195, "Velocity"=w194, "Velocity"=w193, "Velocity"=w192) -> (w187:T40)  [unwired: 1 in]
          n97 = call "Set Target Velocity.vi"("epsilon"=100.0, "Control Mode"=w185, "Input (ft/s)"=w187, "Swerve motors"=w182) -> ("we done yet????!?!?!"=w160:bool)  [unwired: 6 in, 1 out]
          n98 = call "Set Target Position.vi"("conv to ticks?"=TRUE, "Control Mode"=w184, "Input (deg)"=w180, "Swerve motors"=w181) -> ()  [unwired: 7 in, 1 out]
          n99 = And(x=w160, y=w156) -> (x .and. y?=w158:bool)
          n100 = node-c288() -> ()  [unwired: 1 in, 1 out]
        }
        n101 = node-c288(w147) -> ()  [unwired: 1 out]
      }
      frame "Set Schtuff" {
        w236 = 1 ("length")
        n102 = Unbundle(w246) -> ("Translations"=w238:cluster{"x out":dbl, "y out":dbl}[], "Rotations"=w237:cluster{"omega":dbl, "theta":dbl}[])  [unwired: 1 out]
        n103 = Array Subset(array=w237, length=w236) -> (w234:cluster{"omega":dbl, "theta":dbl}[])  [unwired: 1 in]
        n104 = Array Subset(array=w238, length=w236) -> (w235:cluster{"x out":dbl, "y out":dbl}[])  [unwired: 1 in]
        n105 = Array Size(array=w234) -> (size(s)=w240:i32)
        n106 = node-c288() -> (w248:T32)  [unwired: 4 in]
        n107 = timed-loop {
          timing: w248 -> [_]
          timing-out: [_] -> w247
          tunnel: w235 -> [w262]
          tunnel: w234 -> [w261]
          tunnel: w245 -> [w276]
          tunnel: w244 -> [w277]
          tunnel: w241 -> [w263]
          tunnel: w240 -> [w256]
          tunnel: w239 -> [w267]
          i -> [w257]
          stop <- w253 stop-if-true
          w279 = T36 1 items=["PercentOutput"=0, "Position"=1, "Velocity"=2, "Current"=3, "Follower"=5, "MotionProfile"=6, "MotionMagic"=7, "MotionProfileArc"=10, "Disabled"=15] ("Control Mode")
          w280 = T36 2 items=["PercentOutput"=0, "Position"=1, "Velocity"=2, "Current"=3, "Follower"=5, "MotionProfile"=6, "MotionMagic"=7, "MotionProfileArc"=10, "Disabled"=15] ("Control Mode")
          n108 = node-c288() -> ()  [unwired: 1 in, 1 out]
          n109 = Max & Min(x=w256, y=w257) -> (min(x,y)=w254:i32)  [unwired: 1 out]
          n110 = Greater Or Equal?(x=w257, y=w256) -> (x >= y?=w251:bool)
          n111 = Index Array(array=w262, index=w254) -> (element=w260:cluster{"x out":dbl, "y out":dbl})
          n112 = Index Array(array=w261, index=w254) -> (element=w259:cluster{"omega":dbl, "theta":dbl})
          n113 = call "ADIS16470 Read Velocity.vi"("ADIS16470DevRef"=w267) -> ("ADIS16470 Value"=w272:T37)  [unwired: 7 in, 3 out]
          n114 = Unbundle(w272) -> ("ZAngle"=w269:dbl)  [unwired: 2 out]
          n115 = Unbundle(w259) -> ("omega"=w274:dbl, "theta"=w268:dbl)
          n116 = call "ADIS16470 Read Position.vi"("ADIS16470DevRef"=w267) -> ("ADIS16470 Value"=w266:T37)  [unwired: 7 in, 3 out]
          n117 = Unbundle(w260) -> ("x out"=w270:dbl, "y out"=w271:dbl)
          n118 = Unbundle(w266) -> ("YAngle"=w265:dbl)  [unwired: 2 out]
          n119 = Compound Arithmetic op=AND("IMU Correction  2", invert w251) -> (w250:bool)
          n120 = case shown="True" w250 {
            tunnel: w269 -> [_ w300]
            tunnel: w274 -> [w294 w298]
            tunnel: [w294 w297] -> w273
            tunnel: w268 -> [_ w296]
            tunnel: w265 -> [_ w295]
            frame False {
            }
            frame True {
              n121 = call "IMU Correction.vi"("omega"=w298, "Heading Setpoint"=w296, "theta"=w295, "measured angle"=w300) -> ("Difference"=w299:dbl)  [unwired: 7 in]
              n122 = Add(x=w298, y=w299) -> (x+y=w297:dbl)
            }
          }
          n123 = Bundle("x out"=w270, "y out"=w271, "omega"=w273) -> (w278:cluster{"x out":dbl, "y out":dbl, "omega":dbl})  [unwired: 1 in]
          n124 = call "Get Steering Angles.vi"("Input Steering"=w276) -> ("Steering Angles (deg)"=w281:T38)  [unwired: 10 in]
          n125 = call "Inverse Kinematics.vi"("Current Pod Steering (deg)"=w281, "Radii (ft)"=w263, "Target Velocity (ft/s and deg/s)"=w278) -> ("RB Pod Setpoint (ft/s and deg/s)"=w290:cluster{"Velocity":dbl, "Theta":dbl}, "RF Pod Setpoint (ft/s and deg/s)"=w291:cluster{"Velocity":dbl, "Theta":dbl}, "LB Pod Setpoint (ft/s and deg/s)"=w292:cluster{"Velocity":dbl, "Theta":dbl}, "LF Pod Setpoint (ft/s and deg/s)"=w293:cluster{"Velocity":dbl, "Theta":dbl})  [unwired: 2 in, 3 out]
          n126 = Unbundle(w293) -> ("Velocity"=w289:dbl, "Theta"=w285:dbl)
          n127 = Unbundle(w292) -> ("Velocity"=w288:dbl, "Theta"=w284:dbl)
          n128 = Unbundle(w291) -> ("Velocity"=w287:dbl, "Theta"=w283:dbl)
          n129 = Unbundle(w290) -> ("Velocity"=w286:dbl, "Theta"=w282:dbl)
          n130 = Bundle("Theta"=w285, "Theta"=w284, "Theta"=w283, "Theta"=w282) -> (w275:T39)  [unwired: 1 in]
          n131 = Bundle("Velocity"=w289, "Velocity"=w288, "Velocity"=w287, "Velocity"=w286) -> ()  [unwired: 1 in, 1 out]
          n132 = call "Set Target Velocity.vi"("epsilon"=100.0, "Control Mode"=w280, "Input (ft/s)"=cluster{"LF":dbl, "LB":dbl, "RF":dbl, "RB":dbl} {"LF"=0.0, "LB"=0.0, "RF"=0.0, "RB"=0.0} ("Input (deg)"), "Swerve motors"=w277) -> ("we done yet????!?!?!"=w255:bool)  [unwired: 6 in, 1 out]
          n133 = call "Set Target Position.vi"("conv to ticks?"=TRUE, "Control Mode"=w279, "Input (deg)"=w275, "Swerve motors"=w276) -> ()  [unwired: 7 in, 1 out]
          n134 = And(x=w255, y=w251) -> (x .and. y?=w253:bool)
          n135 = node-c288() -> ()  [unwired: 1 in, 1 out]
        }
        n136 = node-c288(w247) -> ()  [unwired: 1 out]
      }
      frame "Calibrate" {
        n137 = call "Get Cancoder Absolute Angles.vi"("Input Cancoders"=w313) -> ("offsets"=w305:cluster{dbl, dbl, dbl, dbl})  [unwired: 10 in]
        "offsets" <- w305
        n138 = Unbundle(w312) -> ("PhoenixMotorControlDevRef"=w311:T15, "PhoenixMotorControlDevRef"=w310:T15, "PhoenixMotorControlDevRef"=w309:T15, "PhoenixMotorControlDevRef"=w308:T15)
        n139 = disable-structure shown="Enabled" {
          disable-tunnel: w312 -> [w327 _]
          disable-tunnel: w311 -> [w326 _]
          disable-tunnel: w310 -> [w325 _]
          disable-tunnel: w309 -> [w324 _]
          disable-tunnel: w308 -> [w323 _]
          disable-tunnel: [w319 _] -> w307
          disable-tunnel: [w317 _] -> w306
          disable-tunnel: w305 -> [w316 _]
          frame Enabled {
            n140 = flat-sequence {
              tunnel: w316 -> [w356]
              tunnel: w326 -> [w340]
              tunnel: w325 -> [w355]
              tunnel: w324 -> [w354]
              tunnel: w323 -> [w353]
              tunnel: [500] -> w333
              tunnel: [w335] -> w332
              tunnel: [w344] -> w331
              tunnel: [w343] -> w330
              tunnel: [w342] -> w329
              tunnel: [w334] -> w328
              tunnel: [w360] -> w320
              tunnel: [w361] -> w321
              tunnel: [w362] -> w322
              tunnel: [w363] -> w318
              tunnel: [w364] -> w317
              tunnel: w333 -> [w364]
              tunnel: w332 -> [w363]
              tunnel: w331 -> [w362]
              tunnel: w330 -> [w361]
              tunnel: w329 -> [w360]
              tunnel: w328 -> [w358]
              tunnel: w327 -> [w357]
              frame #0 {
                # "offsets"
                n141 = Unbundle(w356) -> (w348:dbl, w347:dbl, w346:dbl, w345:dbl)
                n142 = call "Angle Wrapper.vi"("angle in"=w348) -> ("angle out"=w339:dbl)  [unwired: 10 in]
                n143 = call "Angle Wrapper.vi"("angle in"=w347) -> ("angle out"=w338:dbl)  [unwired: 10 in]
                n144 = call "Angle Wrapper.vi"("angle in"=w346) -> ("angle out"=w337:dbl)  [unwired: 10 in]
                n145 = call "Angle Wrapper.vi"("angle in"=w345) -> ("angle out"=w336:dbl)  [unwired: 10 in]
                n146 = call "Degrees To Ticks.vi"("degrees"=w339) -> ("ticks"=w341:dbl)  [unwired: 10 in]
                n147 = call "Degrees To Ticks.vi"("degrees"=w338) -> ("ticks"=w351:dbl)  [unwired: 10 in]
                n148 = call "Degrees To Ticks.vi"("degrees"=w337) -> ("ticks"=w350:dbl)  [unwired: 10 in]
                n149 = call "Degrees To Ticks.vi"("degrees"=w336) -> ("ticks"=w349:dbl)  [unwired: 10 in]
                n150 = call <vilib>:"CTRE_Phoenix_MotorControl_SetSelectedSensorPosition.vi"("New Sensor Position"=w341, "PhoenixMotorControlDevRef"=w340) -> ("PhoenixMotorControlDevRef"=w335:T15)  [unwired: 8 in, 1 out]
                n151 = call <vilib>:"CTRE_Phoenix_MotorControl_SetSelectedSensorPosition.vi"("New Sensor Position"=w351, "PhoenixMotorControlDevRef"=w355) -> ("PhoenixMotorControlDevRef"=w344:T15)  [unwired: 8 in, 1 out]
                n152 = call <vilib>:"CTRE_Phoenix_MotorControl_SetSelectedSensorPosition.vi"("New Sensor Position"=w350, "PhoenixMotorControlDevRef"=w354) -> ("PhoenixMotorControlDevRef"=w343:T15)  [unwired: 8 in, 1 out]
                n153 = call <vilib>:"CTRE_Phoenix_MotorControl_SetSelectedSensorPosition.vi"("New Sensor Position"=w349, "PhoenixMotorControlDevRef"=w353) -> ("PhoenixMotorControlDevRef"=w342:T15)  [unwired: 8 in, 1 out]
                n154 = Bundle("angle out"=w339, "angle out"=w338, "angle out"=w337, "angle out"=w336) -> (w334:T41)  [unwired: 1 in]
              }
              frame #1 {
                w359 = T36 1 items=["PercentOutput"=0, "Position"=1, "Velocity"=2, "Current"=3, "Follower"=5, "MotionProfile"=6, "MotionMagic"=7, "MotionProfileArc"=10, "Disabled"=15] ("Control Mode")
                n155 = call "Set Target Position.vi"("Control Mode"=w359, "Input (deg)"=w358, "Swerve motors"=w357) -> ()  [unwired: 8 in, 1 out]
              }
            }
            n156 = Bundle("PhoenixMotorControlDevRef"=w318, "PhoenixMotorControlDevRef"=w322, "PhoenixMotorControlDevRef"=w321, "PhoenixMotorControlDevRef"=w320) -> (w319:T20)  [unwired: 1 in]
          }
          frame Disabled {
          }
        }
        n157 = disable-structure shown="Disabled" {
          disable-tunnel: w307 -> [w368 _]
          disable-tunnel: w306 -> [w367 _]
          disable-tunnel: [w366 TRUE] -> w314
          frame Disabled {
            n158 = case shown="True" "RESET CANCODERS -- TEST" {
              tunnel: w367 -> [_ w375]
              tunnel: w368 -> [_ w374]
              tunnel: [TRUE w370] -> w366
              frame False {
              }
              frame True {
                n159 = Wait (ms)(milliseconds to wait=w375) -> (millisecond timer value=w373:u32)
                n160 = flat-sequence {
                  tunnel: w374 -> [w380]
                  tunnel: w373 -> [_]
                  tunnel: [1000] -> w372
                  frame #0 {
                    w379 = T36 1 items=["PercentOutput"=0, "Position"=1, "Velocity"=2, "Current"=3, "Follower"=5, "MotionProfile"=6, "MotionMagic"=7, "MotionProfileArc"=10, "Disabled"=15] ("Control Mode")
                    n161 = call "Set Target Position.vi"("Control Mode"=w379, "Input (deg)"=cluster{"LF":dbl, "LB":dbl, "RF":dbl, "RB":dbl} {"LF"=0.0, "LB"=0.0, "RF"=0.0, "RB"=0.0}, "Swerve motors"=w380) -> ()  [unwired: 8 in, 1 out]
                  }
                }
                n162 = Wait (ms)(milliseconds to wait=w372) -> (millisecond timer value=w371:u32)
                n163 = flat-sequence {
                  tunnel: w371 -> [_]
                  tunnel: [TRUE] -> w370
                  frame #0 {
                  }
                }
              }
            }
          }
          frame Enabled {
          }
        }
      }
      frame "Reserve" {
        w384 = T36 2 items=["PercentOutput"=0, "Position"=1, "Velocity"=2, "Current"=3, "Follower"=5, "MotionProfile"=6, "MotionMagic"=7, "MotionProfileArc"=10, "Disabled"=15] ("Control Mode")
        w388 = -1.0  # Infinite
        n164 = disable-structure shown="Enabled" {
          disable-tunnel: w383 -> [w390 _]
          frame Enabled {
            w389 = T36 0 items=["PercentOutput"=0, "Position"=1, "Velocity"=2, "Current"=3, "Follower"=5, "MotionProfile"=6, "MotionMagic"=7, "MotionProfileArc"=10, "Disabled"=15] ("Control Mode")
            n165 = call "Set Target Position.vi"("Control Mode"=w389, "Input (deg)"=cluster{"LF":dbl, "LB":dbl, "RF":dbl, "RB":dbl} {"LF"=0.0, "LB"=0.0, "RF"=0.0, "RB"=0.0}, "Swerve motors"=w390) -> ()  [unwired: 8 in, 1 out]
          }
          frame Disabled {
          }
        }
        n166 = call "Set Target Velocity.vi"("epsilon"=1.0, "Control Mode"=w384, "Input (ft/s)"=cluster{"LF":dbl, "LB":dbl, "RF":dbl, "RB":dbl} {"LF"=0.0, "LB"=0.0, "RF"=0.0, "RB"=0.0} ("Velocities"), "Swerve motors"=w385) -> ()  [unwired: 6 in, 2 out]
      }
    }
    n167 = call "Drive Check for New Command.vi"("input cluster"=w28, "Wait time (ms)"=w42, "Finished?"=w41) -> ("Completion"=w44:T7, "Subsystem Name"=w38:string, "Current Command"=w39:T3, "Initial Trace String"=w40:string, "Next Command"=w43:T42)  [unwired: 4 in]
    n168 = case shown="\"Successful\", \"Aborted\"" w44 {
      selector: w44 -> [_ w60]
      tunnel: w40 -> [_ w57]
      tunnel: w39 -> [_ w58]
      tunnel: w38 -> [_ w55]
      frame "Incomplete", Default {
        # "Continuing current command"
      }
      frame "Successful", "Aborted" {
        # "Report and setup for next command"
        n169 = Unbundle By Name(w58) -> ("Trans Vel.x"=w54:dbl, "Trans Vel.y"=w53:dbl, "Rot Vel.omega"=w52:dbl)
        n170 = disable-structure shown="Disabled" {
          disable-tunnel: w54 -> [w71 _]
          disable-tunnel: w53 -> [w68 _]
          disable-tunnel: w52 -> [w67 _]
          frame Disabled {
            w63 = TRUE ("use timestamp? (F)")
            w65 = "Drive" ("subsystem")
            n171 = global read "Robot Global Data.vi" "logger"() -> (w73:T43)
            n172 = call "numlock write.vim"("tag"="vx", "use timestamp? (T)"=w63, "subsystem"=w65, "data"=w71, "logger"=w73) -> ("error out"=w62:errorcluster, "logger out"=w70:T43)  [unwired: 5 in]
            n173 = call "numlock write.vim"("tag"="vy", "use timestamp? (T)"=w63, "subsystem"=w65, "error in (no error)"=w62, "data"=w68, "logger"=w70) -> ("error out"=w61:errorcluster, "logger out"=w66:T43)  [unwired: 4 in]
            n174 = call "numlock write.vim"("tag"="omega", "use timestamp? (T)"=w63, "subsystem"=w65, "error in (no error)"=w61, "data"=w67, "logger"=w66) -> ()  [unwired: 4 in, 2 out]
          }
          frame Enabled {
          }
        }
        n175 = Format Into String(format string="TX %.1f, TY %.1f, ROT %.1f", initial string=w57, w54, w53, w52) -> (resulting string=w56:string)  [unwired: 1 in, 1 out]
        "Current\nCmd" <- w56
        n176 = call <vilib>:"Trace Results.vi"("Status of previous command"=w60, "Description"=w56, "Subsystem"=w55) -> ()  [unwired: 9 in]
      }
    }
  }
  n177 = while {
    tunnel: w18 -> [w393]
    stop <- FALSE stop-if-true
    n178 = call "Drive Controller Interactive Check.vi"("Interactive Command In"="Interactive Values", "Default Command"=w393, "Buttons"="Buttons") -> ("Interactive Command Out"=w395:T3, "Trace String"=w396:string, "Schedule"=w397:bool)  [unwired: 6 in]
    n179 = case shown="False" w397 {
      tunnel: [w405 w412] -> w398
      tunnel: [w404 _] -> _
      tunnel: w396 -> [_ w410]
      tunnel: w395 -> [_ w409]
      frame False {
        n180 = Tick Count (ms)() -> (millisecond timer value=w408:u32)
        n181 = call "Read Drive Operation.vi"() -> ("Command Info"=w402:T10, "SubSystem Data"=w401:T3)  [unwired: 9 in, 1 out]
        n182 = Unbundle(w401) -> ("Operation"=w406:T4, "Trans Vel"=w403:cluster{"x":dbl, "y":dbl})  [unwired: 4 out]
        n183 = Unbundle(w402) -> ("Status"=w405:T7)  [unwired: 2 out]
        n184 = Subtract(x=w408, y=w406) -> (x-y=w407:u32)
        n185 = Bundle(w407, "Trans Vel"=w403) -> (w404:T44)  [unwired: 1 in]
      }
      frame True {
        n186 = call "Drive Command Helper.vi"("Description"=w410, "SubSystem Data"=w409) -> ("Command Info Out"=w411:T10)  [unwired: 7 in, 2 out]
        n187 = Unbundle(w411) -> ("Status"=w412:T7)  [unwired: 2 out]
      }
    }
    "Status" <- w398
    n188 = Wait (ms)(milliseconds to wait=u32 20) -> ()  [unwired: 1 out]
  }
